vi "All Variant to strings.vi"(3 "Error in":errorcluster caption="错误输入", 5 "Variant input":variant[](array[variant])) -> (0 "Error out":errorcluster caption="错误输出", 1 "Var Out":string[](array[string]))   [LabVIEW 2014]
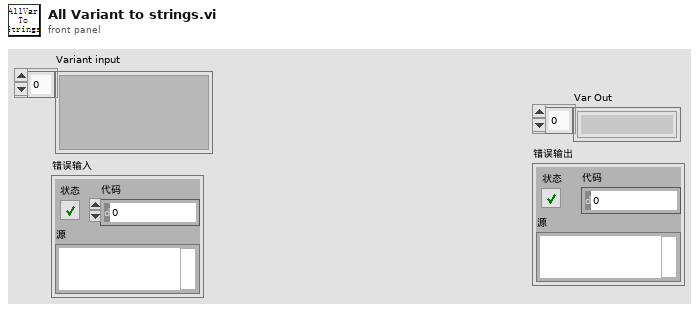
[diagram p1: front panel]
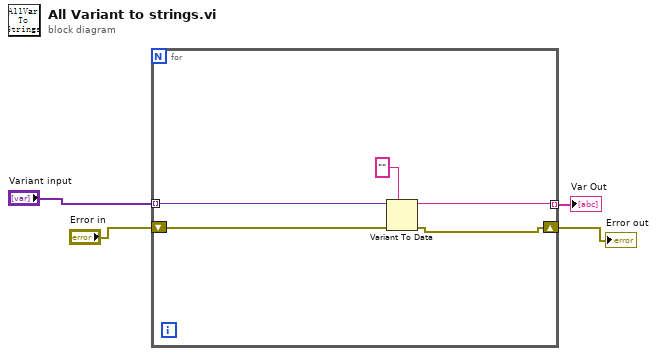
[diagram p0: block diagram]
diagram:
  n1 = for {
    tunnel: "Variant input" -> [w9] mode=indexing
    tunnel: [w7] -> w3 mode=indexing
    shift-right: [w5] -> w1
    shift-left: "Error in" -> [w6]
    n2 = Variant To Data(error in=w6, type="", Variant=w9) -> (data=w7:string, error out=w5:errorcluster)
  }
  "Var Out" <- w3
  "Error out" <- w1
